vi "Channel Probe.vi"(2 "channelOp":T2=enum."Publish", 3 "tagData in":T3) -> (1 "tagData out":T3)   [LabVIEW 2020, in "Flex.lvlib"]
doc: "Displays the status of the channel as the channel is modified by the various endpoints and gives the user ways to pause the application using the channel."
uses:
  Flex.lvlib
  TagData.lvclass
  Element.ctl
  ChannelOp.ctl
  Channel Data.ctl
panel:
  in  "Single Step":bool
  out "Tag Name":string="<Unnamed>"
  in  "Sequence Number To Match":i32
  in  "Pause when Sequence Number matches":bool
  in  "Value To Match":T1
  in  "Pause when Tag Value matches":bool
  in  "Pause when aborted":bool
  in  "Step To Next Write":bool
  in  "Play":bool
  out "Aborted?":bool
  out "Sequence Number":i32
  out "Tag Name":string
  out "Tag Value":T1
  in  "Pause":bool
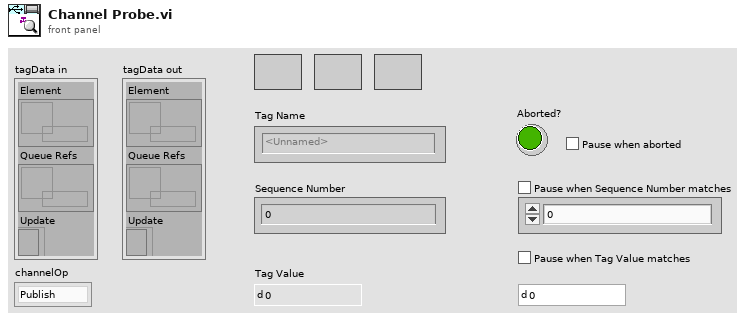
[diagram p1: front panel]
types:
  T1 = typedef "Flex.lvlib/Element.ctl" = dbl
  T2 = typedef "Flex.lvlib/ChannelOp.ctl" = enum16{"Init", "Publish", "Latest", "Next", "Close", "Probe"}
  T3 = typedef "Flex.lvlib/Channel Data.ctl" = cluster{"Element":refnum<data-value>, "Queue Refs":refnum<data-value>, "Update":refnum<k4>}
  T4 = enum32{"Invalid", "Standard", "Closed", "Hidden", "Minimized", "Maximized"}
  T5 = typedef "LVPointTypeDef.ctl" = cluster{"Horizontal":i16, "Vertical":i16}
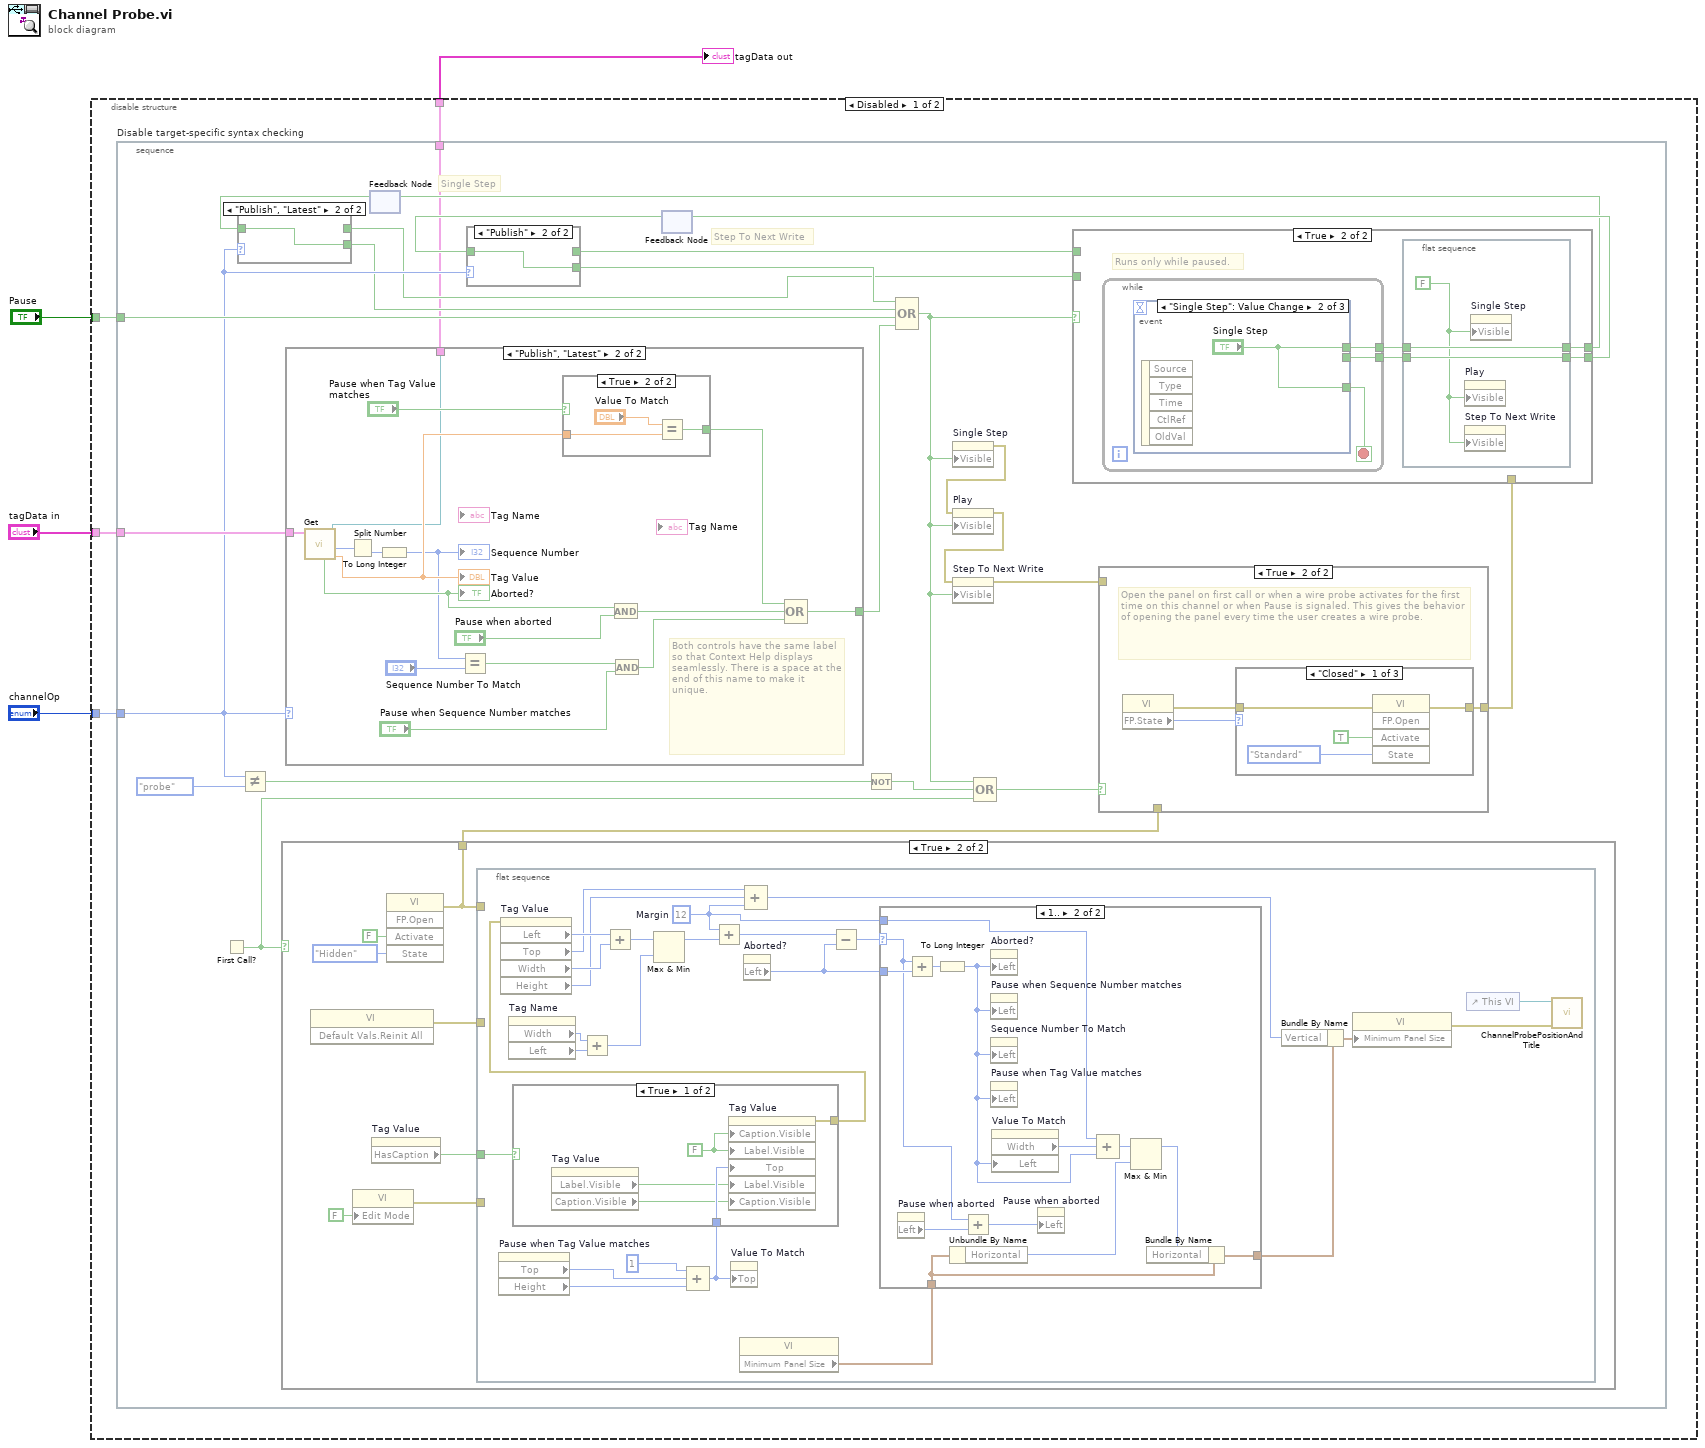
[diagram p0: block diagram]
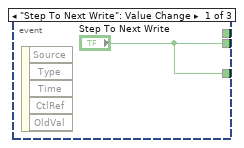
[diagram p5: hidden frame]
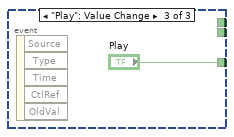
[diagram p6: hidden frame]
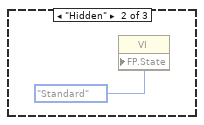
[diagram p10: hidden frame]
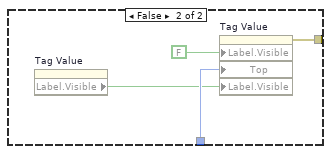
[diagram p13: hidden frame]
diagram:
  n1 = disable-structure shown="Disabled" {
    disable-tunnel: "tagData in" -> [w8 w135]
    disable-tunnel: "Pause" -> [w7 _]
    disable-tunnel: "channelOp" -> [w6 _]
    disable-tunnel: [w5 w135] -> w1
    frame Disabled {
      n2 = stacked-sequence "Disable target-specific syntax checking" {
        tunnel: w8 -> [w32]
        tunnel: w7 -> [w25]
        tunnel: w6 -> [w15]
        tunnel: [w9] -> w5
        frame #0 {
          # "Step To Next Write"
          # "Single Step"
          n3 = First Call?() -> (First Call?: T/F=w30:bool)
          n4 = Not Equal?(x=w15, y=enum16{"init", "write", "read", "probe"}."probe" ("channelOp 2")) -> (x != y?=w27:bool)
          n5 = case shown="True" w30 {
            tunnel: [_ w81] -> w18
            frame False {
            }
            frame True {
              n6 = invoke class="VI" method="Default Vals.Reinit All"() -> (error out=w82:errorcluster)  [unwired: 3 in, 2 out]
              n7 = property class="VI"("Edit Mode"=FALSE ("Edit Mode On Open")) -> (error out=w83:errorcluster)  [unwired: 2 in, 1 out]
              n8 = property on="Tag Value" class="DigNum (strict)"() -> ("HasCaption"=w80:bool)  [unwired: 2 in, 2 out]
              n9 = invoke class="VI" method="FP.Open"("Activate"=FALSE ("Activate?"), "State"=T4."Hidden") -> (error out=w81:errorcluster)  [unwired: 3 in, 4 out]
              n10 = flat-sequence {
                tunnel: w81 -> [_]
                tunnel: w83 -> [_]
                tunnel: w82 -> [_]
                tunnel: w80 -> [w95]
                frame #0 {
                  w93 = 12  # Margin
                  n11 = property on="Pause when Tag Value matches" class="Bool (strict)"() -> ("Top"=w103:i32, "Height"=w102:u32)  [unwired: 2 in, 2 out]
                  n12 = property on="Tag Name" class="Str"() -> ("Width"=w91:u32, "Left"=w90:i32)  [unwired: 2 in, 2 out]
                  n13 = Add(x=w91, y=w90) -> (x+y=w88:u32)
                  n14 = Compound Arithmetic op=ADD(u32 1 ("value"), w103, w102) -> (w101:u32)
                  n15 = case shown="True" w95 {
                    tunnel: w101 -> [w116 w120]
                    tunnel: [w115 w119] -> w99
                    frame True {
                      w112 = FALSE ("Label.Visible")
                      n16 = property on="Tag Value" class="DigNum (strict)"() -> ("Label.Visible"=w114:bool, "Caption.Visible"=w113:bool)  [unwired: 2 in, 2 out]
                      n17 = property on="Tag Value" class="DigNum (strict)"("Caption.Visible"=w112, "Label.Visible"=w112, "Top"=w116, "Label.Visible"=w114, "Caption.Visible"=w113) -> (error out=w115:errorcluster)  [unwired: 2 in, 1 out]
                    }
                    frame False {
                      n18 = property on="Tag Value" class="DigNum (strict)"() -> ("Label.Visible"=w117:bool)  [unwired: 2 in, 2 out]
                      n19 = property on="Tag Value" class="DigNum (strict)"("Label.Visible"=FALSE, "Top"=w120, "Label.Visible"=w117) -> (error out=w119:errorcluster)  [unwired: 2 in, 1 out]
                    }
                  }
                  n20 = property on="Tag Value" class="DigNum (strict)"(error in=w99) -> ("Left"=w111:i32, "Top"=w106:i32, "Width"=w110:u32, "Height"=w105:u32)  [unwired: 1 in, 2 out]
                  n21 = Add(x=w111, y=w110) -> (x+y=w89:u32)
                  n22 = Max & Min(x=w89, y=w88) -> (max(x,y)=w87:u32)  [unwired: 1 out]
                  n23 = Add(x=w93, y=w87) -> (x+y=w109:u32)
                  n24 = property on="Value To Match" class="DigNum (strict)"("Top"=w101) -> ()  [unwired: 2 in, 2 out]
                  n25 = property class="VI"() -> ("Minimum Panel Size"=w94:T5)  [unwired: 2 in, 2 out]
                  n26 = property on="Aborted?" class="Bool (strict)"() -> ("Left"=w107:i32)  [unwired: 2 in, 2 out]
                  n27 = Compound Arithmetic op=ADD(w106, w105, w93) -> (w104:u32)
                  n28 = Subtract(x=w109, y=w107) -> (x-y=w108:u32)
                  n29 = case shown="1.." w108 {
                    selector: w108 -> [_ w132]
                    tunnel: w107 -> [_ w134]
                    tunnel: w94 -> [w121 w124]
                    tunnel: w93 -> [_ w127]
                    tunnel: [w121 w122] -> w92
                    frame Default {
                    }
                    frame 1.. {
                      n30 = property on="Pause when aborted" class="Bool (strict)"() -> ("Left"=w133:i32)  [unwired: 2 in, 2 out]
                      n31 = Add(x=w132, y=w134) -> (x+y=w130:u32)
                      n32 = To Long Integer(number=w130) -> (32bit integer=w128:i32)
                      n33 = Unbundle By Name(w124) -> ("Horizontal"=w125:i16)
                      n34 = Add(x=w132, y=w133) -> (x+y=w131:u32)
                      n35 = property on="Aborted?" class="Bool (strict)"("Left"=w128) -> ()  [unwired: 2 in, 2 out]
                      n36 = property on="Pause when Sequence Number matches" class="Bool (strict)"("Left"=w128) -> ()  [unwired: 2 in, 2 out]
                      n37 = property on="Sequence Number To Match" class="DigNum (strict)"("Left"=w128) -> ()  [unwired: 2 in, 2 out]
                      n38 = property on="Pause when Tag Value matches" class="Bool (strict)"("Left"=w128) -> ()  [unwired: 2 in, 2 out]
                      n39 = property on="Value To Match" class="DigNum (strict)"("Left"=w128) -> ("Width"=w129:u32)  [unwired: 2 in, 2 out]
                      n40 = property on="Pause when aborted" class="Bool (strict)"("Left"=w131) -> ()  [unwired: 2 in, 2 out]
                      n41 = Compound Arithmetic op=ADD(w127, w129, w128) -> (w126:u32)
                      n42 = Max & Min(x=w126, y=w125) -> (max(x,y)=w123:u32)  [unwired: 1 out]
                      n43 = Bundle By Name(cluster=w124, "Horizontal"=w123) -> (w122:T5)
                    }
                  }
                  n44 = Bundle By Name(cluster=w92, "Vertical"=w104) -> (w98:T5)
                  n45 = property class="VI"("Minimum Panel Size"=w98) -> (error out=w97:errorcluster)  [unwired: 2 in, 1 out]
                  n46 = control-ref of="This VI"() -> (w96:refnum<vi>)
                  n47 = call <resource>:"ChannelProbePositionAndTitle.vi"("error in (no error)"=w97, "VI in"=w96) -> ()  [unwired: 8 in, 2 out]
                }
              }
            }
          }
          n48 = case shown="\"Publish\", \"Latest\"" w15 {
            tunnel: w32 -> [w52 w68]
            tunnel: [_ w57] -> w26
            tunnel: [w52 w55] -> w9
            frame Default {
            }
            frame "Publish", "Latest" {
              # "Both controls have the same label so that Context Help displays seamlessly. There is a space at the end of this name to make it unique."
              n49 = call "Get.vi"("TagData in"=w68) -> ("element"=w59:T1, "sequence"=w56:u64, "TagData out"=w55:refnum<class "TagData.lvclass">, "aborted?"=w65:bool)  [unwired: 6 in, 1 out]
              "Tag Value" <- w59
              "Aborted?" <- w65
              n50 = Split Number(x=w56) -> (lo(x)=w54:u32)  [unwired: 1 out]
              n51 = To Long Integer(number=w54) -> (32bit integer=w53:i32)
              "Sequence Number" <- w53
              n52 = Equal?(x=w53, y="Sequence Number To Match") -> (x = y?=w63:bool)
              n53 = case shown="True" "Pause when Tag Value matches" {
                tunnel: w59 -> [_ w70]
                tunnel: [_ w69] -> w58
                frame False {
                }
                frame True {
                  n54 = Equal?(x="Value To Match", y=w70) -> (x = y?=w69:bool)
                }
              }
              n55 = And(x=w65, y="Pause when aborted") -> (x .and. y?=w64:bool)
              n56 = And(x=w63, y="Pause when Sequence Number matches") -> (x .and. y?=w61:bool)
              n57 = Compound Arithmetic op=OR(w58, w64, w61) -> (w57:bool)
            }
          }
          n58 = feedback #1() -> (w16:bool)  [unwired: 1 in]
          n59 = case shown="\"Publish\", \"Latest\"" w15 {
            tunnel: w16 -> [w33 w34]
            tunnel: [_ w34] -> w13
            tunnel: [w33 _] -> w12
            frame Default {
            }
            frame "Publish", "Latest" {
            }
          }
          n60 = feedback #2() -> (w23:bool)  [unwired: 1 in]
          n61 = case shown="\"Publish\"" w15 {
            tunnel: w23 -> [w35 w36]
            tunnel: [_ w36] -> w14
            tunnel: [w35 _] -> w22
            frame Default {
            }
            frame "Publish" {
            }
          }
          n62 = Not(x=w27) -> (.not. x?=w31:bool)
          n63 = Compound Arithmetic op=OR(w14, w13, w25, w26) -> (w11:bool)
          n64 = property on="Single Step" class="Bool"("Visible"=w11) -> (error out=w10:errorcluster)  [unwired: 2 in, 1 out]
          n65 = property on="Play" class="Bool"(error in=w10, "Visible"=w11) -> (error out=w21:errorcluster)  [unwired: 1 in, 1 out]
          n66 = property on="Step To Next Write" class="Bool"(error in=w21, "Visible"=w11) -> (error out=w20:errorcluster)  [unwired: 1 in, 1 out]
          n67 = Compound Arithmetic op=OR(w11, w31, w30) -> (w29:bool)
          n68 = case shown="True" w29 {
            tunnel: w20 -> [_ _]
            tunnel: [_ w72] -> w19
            tunnel: w18 -> [_ _]
            frame False {
            }
            frame True {
              # "Open the panel on first call or when a wire probe activates for the first time on this channel or when Pause is signaled. This gives the behavior of opening the panel every time the user creates a wire probe."
              n69 = property class="VI"() -> (error out=w73:errorcluster, "FP.State"=w74:T4)  [unwired: 2 in, 1 out]
              n70 = case shown="\"Closed\"" w74 {
                tunnel: w73 -> [w78 _ _]
                tunnel: [w75 _ _] -> w72
                frame "Closed" {
                  n71 = invoke class="VI" method="FP.Open"(error in=w78, "Activate"=TRUE ("Activate?"), "State"=T4."Standard") -> (error out=w75:errorcluster)  [unwired: 2 in, 4 out]
                }
                frame "Hidden" {
                  n72 = property class="VI"("FP.State"=T4."Standard" ("Front Panel Window:State")) -> ()  [unwired: 2 in, 2 out]
                }
                frame Default {
                }
              }
            }
          }
          n73 = case shown="True" w11 {
            tunnel: [w38 w42] -> w24
            tunnel: w22 -> [w38 _]
            tunnel: w19 -> [_ _]
            tunnel: [w37 w40] -> w17
            tunnel: w12 -> [w37 _]
            frame False {
            }
            frame True {
              # "Runs only while paused."
              n74 = while {
                tunnel: [w48] -> w41
                tunnel: [w46] -> w39
                stop <- w47 stop-if-true
                n75 = event shown="[1] \"Single Step\": Value Change" {
                  selector: _ -> [_ _ _]
                  dyn-events: _ -> [_ _ _]
                  timeout: _ -> [_ _ _]
                  tunnel: ["Step To Next Write" _ _] -> w48
                  tunnel: ["Step To Next Write" "Single Step" "Play"] -> w47
                  tunnel: [_ "Single Step" _] -> w46
                  event "Step To Next Write": Value Change {
                    n76 = event-data() -> ()  [unwired: 1 in, 5 out]
                  }
                  event "Single Step": Value Change {
                    n77 = event-data() -> ()  [unwired: 1 in, 5 out]
                  }
                  event "Play": Value Change {
                    n78 = event-data() -> ()  [unwired: 1 in, 5 out]
                  }
                }
              }
              n79 = flat-sequence {
                tunnel: [w45] -> w42
                tunnel: w41 -> [w45]
                tunnel: [w44] -> w40
                tunnel: w39 -> [w44]
                frame #0 {
                  w43 = FALSE ("Pause")
                  n80 = property on="Play" class="Bool"("Visible"=w43) -> ()  [unwired: 2 in, 2 out]
                  n81 = property on="Step To Next Write" class="Bool"("Visible"=w43) -> ()  [unwired: 2 in, 2 out]
                  n82 = property on="Single Step" class="Bool"("Visible"=w43) -> ()  [unwired: 2 in, 2 out]
                }
              }
            }
          }
          n83 = feedback-in #1(w17) -> ()
          n84 = feedback-in #2(w24) -> ()
        }
      }
    }
    frame Enabled {
    }
  }
  "tagData out" <- w1
